vi "Get Module Main VI Information.vi"(8 "error in (no error)":errorcluster) -> (0 "error out":errorcluster, 1 "Execution State":T1(ring), 2 "Is Module Running?":bool, 3 "Module Main VI":refnum<vi>)   [LabVIEW 2019, in "Server.lvlib"]
doc: "Return information about the module main VI, including its VI reference, its execution state enum, and a Boolean value indicating whether or not it is running.\n_____\nBased on Delacor QMH Project Template 4.2.1.64."
uses:
  Server.lvlib
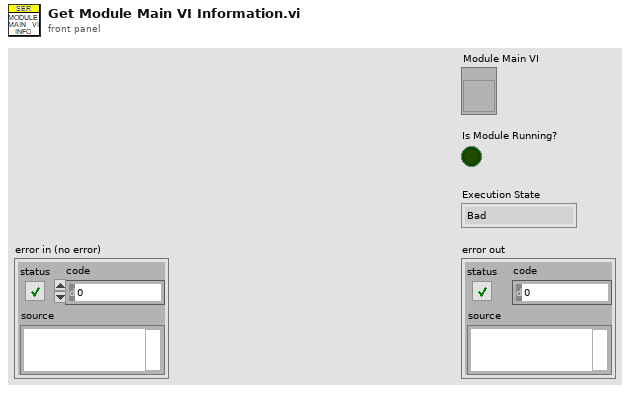
[diagram p1: front panel]
types:
  T1 = enum32{"Bad", "Idle", "Run top level", "Running"}
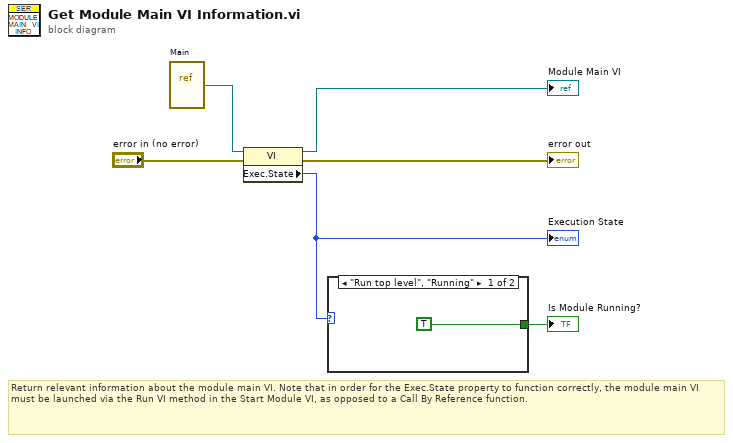
[diagram p0: block diagram]
diagram:
  # "Return relevant information about the module main VI. Note that in order for the Exec.State property to function correctly, the module main VI must be launched via the Run VI method in the Start Module VI, as opposed to a Call By Reference function."
  n1 = vi-ref "Main.vi"() -> (w3:refnum<vi>)
  n2 = property class="VI"(reference=w3, error in="error in (no error)") -> (reference out=→"Module Main VI":refnum<vi>, error out=→"error out":errorcluster, "Exec.State"=w2:T1)
  "Execution State" <- w2
  n3 = case shown="\"Run top level\", \"Running\"" w2 {
    tunnel: [TRUE _] -> w1
    frame "Run top level", "Running" {
    }
    frame "Bad", "Idle" {
    }
  }
  "Is Module Running?" <- w1
